vi "SaveDataFast.vi"(7 "Header In":T1 {"Compression Parameters"."% taper" min=50 max=1000 format="%.2f"; "Compression Parameters"."F2 (MHz)" format="%.3f"; "Compression Parameters"."F1 (MHz)" format="%.3f"; "Scan Settings"."prf (kHz)" format="%.2f"; "Therapy Parameters"."Therapy amplitude (mV)" min=50 max=1000 format="%.2f"; "Therapy Parameters"."Time on (s)" format="%.3f"; "Therapy Parameters"."Theraputic Freq (MHz)" format="%.3f"; "Patient Info"."Race" items=["Am Ind or Alaska", "Asian", "Hawaiian, Pac Isl", "Black or Afr Amer", "White", "more than one race", "unknown"]; "Patient Info"."Ethnicty 2" items=["Hispanic", "Non-Hispanic", "unknown"]; "Patient Info"."LOS" items=["1", "2", "3", "4", "5"]; "Patient Info"."PSA" format="%.1f"; "Scan Info"."delay" format="%.2f"; "Scan Info"."pivot distance" format="%.2f"; "Scan Info"."sector scan angle" format="%.2f"; "Tranducer Info"."bandwidth" format="%.2f"; "Tranducer Info"."center freq" format="%.2f"; "Tranducer Info"."start freq" format="%.2f"}, 8 "error in (no error)":errorcluster, 9 "Save?":bool, 10 "Data Array":dbl[][](array[numeric]), 11 "File Name and Path":path) -> (0 "error out":errorcluster)   [LabVIEW 2022 SP3]
uses:
  Header.ctl
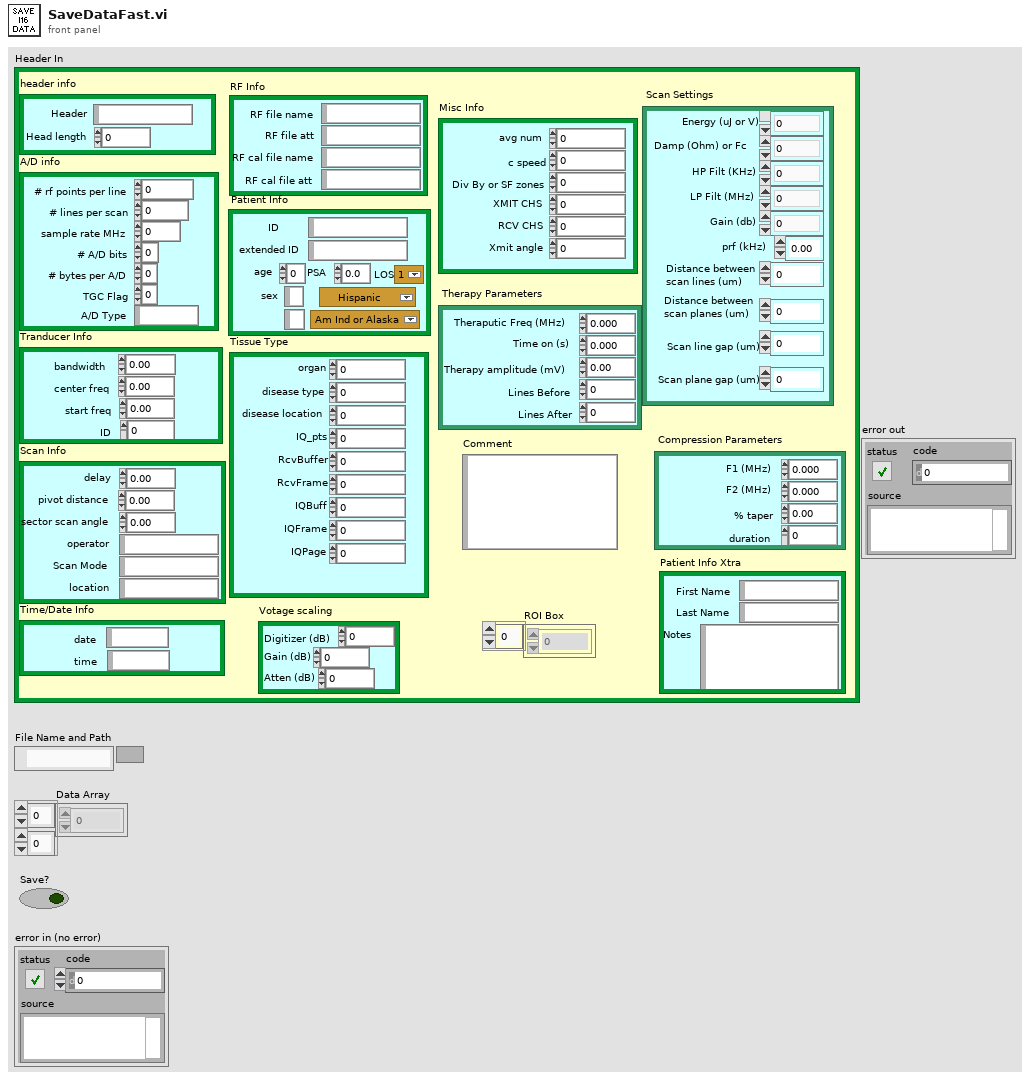
[diagram p1: front panel]
types:
  T1 = typedef "Header.ctl" = cluster{"header info":cluster{"Header":string, "Head length":i16}, "A/D info":cluster{"# rf points per line":u16, "# lines per scan":u16, "sample rate MHz":u16, "# A/D bits":i16, "# bytes per A/D":u16, "TGC Flag":u16, "A/D Type":string}, "Tranducer Info":cluster{"bandwidth":sgl, "center freq":sgl, "start freq":sgl, "ID":i32}, "Scan Info":cluster{"delay":sgl, "pivot distance":sgl, "sector scan angle":sgl, "operator":string, "Scan Mode":string, "location":string}, "Time/Date Info":cluster{"date":string, "time":string}, "RF Info":cluster{"RF file name":string, "RF file att":string, "RF cal file name":string, "RF cal file att":string}, "Patient Info":cluster{"ID":string, "extended ID":string, "age":u16, "sex":string, "previously\nscanned":string, "PSA":sgl, "LOS":u8, "Ethnicty 2":u8, "Race":u8}, "Tissue Type":cluster{"organ":i16, "disease type":i16, "disease location":i16, "IQ_pts":u16, "RcvBuffer":u8, "RcvFrame":u16, "IQBuff":u8, "IQFrame":u16, "IQPage":u8}, "Votage scaling":cluster{"Digitizer (dB)":sgl, "Gain (dB)":sgl, "Atten (dB)":sgl}, "Comment":string, "Misc Info":cluster{"avg num":u16, "c speed":i16, "Div By or SF zones":i16, "XMIT CHS":u8, "RCV CHS":u8, "Xmit angle":sgl}, "Therapy Parameters":cluster{"Theraputic Freq (MHz)":sgl, "Time on (s)":sgl, "Therapy amplitude (mV)":sgl, "Lines Before":u16, "Lines After":u16}, "Scan Settings":cluster{"Energy (uJ or V)":u8, "Damp (Ohm) or Fc":u8, "HP Filt (KHz)":u8, "LP Filt (MHz)":u8, "Gain (db)":u8, "prf (kHz)":sgl, "Distance between\nscan lines (um)":u16, "Distance between\nscan planes (um)":u16, "Scan line gap (um)":sgl, "Scan plane gap (um)":sgl}, "Compression Parameters":cluster{"F1 (MHz)":sgl, "F2 (MHz)":sgl, "% taper":sgl, "duration":sgl}, "Patient Info Xtra":cluster{"First Name":string, "Last Name":string, "Notes":string}, "ROI Box":u16[]}
  T2 = enum16{"big-endian, network order", "native, host order", "little-endian"}
  T3 = enum16{"open", "replace", "create", "open or create", "replace or create", "replace or create with confirmation"}
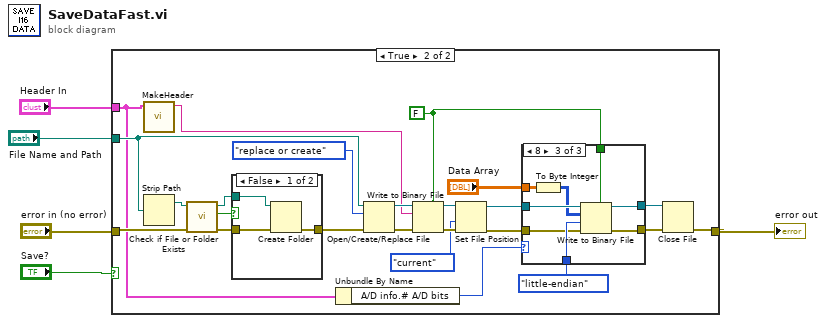
[diagram p0: block diagram]
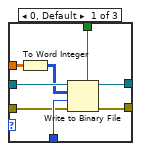
[diagram p3: hidden frame]
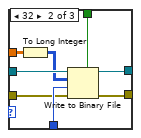
[diagram p4: hidden frame]
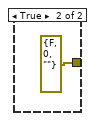
[diagram p5: hidden frame]
diagram:
  n1 = case shown="True" "Save?" {
    tunnel: "Header In" -> [_ w8]
    tunnel: "File Name and Path" -> [_ w13]
    tunnel: "error in (no error)" -> [w6 w12]
    tunnel: [w6 w18] -> w2
    frame False {
    }
    frame True {
      w10 = FALSE ("prepend array or string size? (T)")
      n2 = call "MakeHeader.vi"("Header In"=w8) -> ("Header String"=w19:string)  [unwired: 6 out]
      n3 = Strip Path(path=w13) -> (stripped path=w14:path)  [unwired: 1 out]
      n4 = call <vilib>:"Check if File or Folder Exists.vi"("error in (no error)"=w12, "path"=w14) -> ("error out"=w17:errorcluster, "file or folder exists?"=w15:bool, "dup path"=w16:path)  [unwired: 7 in]
      n5 = case shown="False" w15 {
        tunnel: w17 -> [w57 _]
        tunnel: w16 -> [w56 _]
        tunnel: [w55 errorcluster {"status"=FALSE, "code"=0, "source"=""} ("error out")] -> w11
        frame False {
          n6 = Create Folder(path (use dialog)=w56, error in=w57) -> (error out=w55:errorcluster)  [unwired: 1 in, 2 out]
        }
        frame True {
        }
      }
      n7 = Unbundle By Name(w8) -> ("A/D info.# A/D bits"=w7:i16)
      n8 = Open/Create/Replace File(file path (use dialog)=w13, error in=w11, operation (0:open)=T3."replace or create") -> (refnum out=w26:refnum<file>, error out=w27:errorcluster)  [unwired: 4 out]
      n9 = Write to Binary File(file (use dialog)=w26, data=w19, error in=w27, 5:w10) -> (refnum out=w24:refnum<file>, error out=w25:errorcluster)  [unwired: 3 out]
      n10 = Set File Position(refnum=w24, from (0:start)=enum16{"start", "end", "current"}."current" ("pos mode (0:2)"), error in=w25) -> (refnum out=w28:refnum<file>, error out=w29:errorcluster)  [unwired: 1 out]
      n11 = case shown="8" w7 {
        tunnel: T2."little-endian" ("byte order (0:big-endian, network order)") -> [w38 w46 w54]
        tunnel: w10 -> [w37 w45 w53]
        tunnel: w29 -> [w36 w44 w52]
        tunnel: w28 -> [w35 w43 w51]
        tunnel: [w34 w42 w50] -> w22
        tunnel: [w33 w41 w49] -> w21
        tunnel: "Data Array" -> [w32 w40 w48]
        frame 0, Default {
          n12 = To Word Integer(number=w32) -> (16bit integer=w31:i16[][])
          n13 = Write to Binary File(file (use dialog)=w35, data=w31, error in=w36, 5:w37, 9:w38) -> (refnum out=w34:refnum<file>, error out=w33:errorcluster)  [unwired: 2 out]
        }
        frame 32 {
          n14 = To Long Integer(number=w40) -> (32bit integer=w39:i32[][])
          n15 = Write to Binary File(file (use dialog)=w43, data=w39, error in=w44, 5:w45, 9:w46) -> (refnum out=w42:refnum<file>, error out=w41:errorcluster)  [unwired: 2 out]
        }
        frame 8 {
          n16 = To Byte Integer(number=w48) -> (8bit integer=w47:i8[][])
          n17 = Write to Binary File(file (use dialog)=w51, data=w47, error in=w52, 5:w53, 9:w54) -> (refnum out=w50:refnum<file>, error out=w49:errorcluster)  [unwired: 2 out]
        }
      }
      n18 = Close File(refnum=w22, error in=w21) -> (error out=w18:errorcluster)  [unwired: 1 out]
    }
  }
  "error out" <- w2
